vi "FTW-Messenger-Actor-Request.vi"(0 "Messenger":refnum<class "FTW-Messenger-Actor.lvclass">, 5 "Parameter":string, 7 "Payload":variant, 11 "error in":errorcluster) -> (4 "Messenger out":refnum<class "FTW-Messenger-Actor.lvclass">, 15 "error out":errorcluster)   [LabVIEW 2013, in "FTW-Messenger-Actor.lvclass"]
uses:
  FTW-Messenger-Actor.lvclass
  Message.Actor/FTW-Message-Actor.lvclass
  Messenger/FTW-Messenger.lvclass
panel:
  # "Inputs"
  # "Outputs"
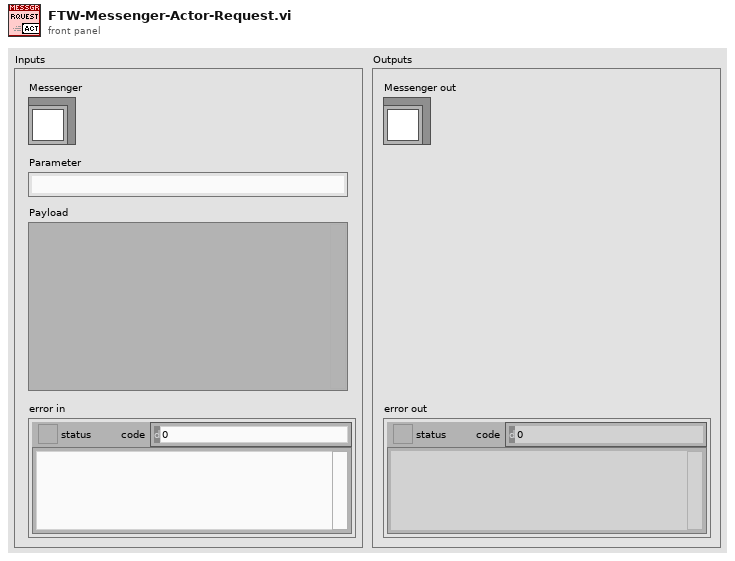
[diagram p1: front panel]
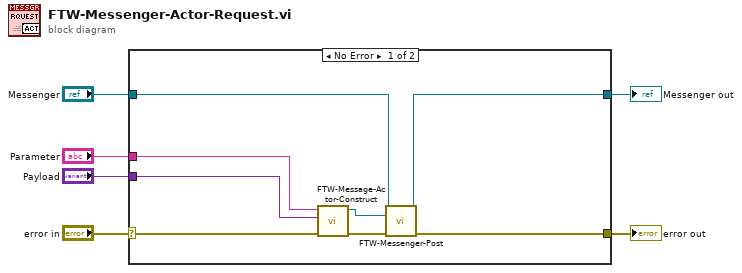
[diagram p0: block diagram]
diagram:
  n1 = case shown="No Error" "error in" {
    selector: "error in" -> [w11 w16]
    tunnel: [w12 w16] -> w5
    tunnel: [w13 w15] -> w6
    tunnel: "Messenger" -> [w14 w15]
    tunnel: "Parameter" -> [w9 _]
    tunnel: "Payload" -> [w8 _]
    frame No Error {
      n2 = call "FTW-Message-Actor-Construct.vi"("error in"=w11, "Payload"=w8, "Parameter"=w9) -> ("error out"=w10:errorcluster, "Actor Message"=w7:refnum<class "FTW-Message-Actor.lvclass">)  [unwired: 7 in]
      n3 = call "FTW-Messenger-Post.vi"("Messenger"=w14, "Message"=w7, "error in"=w10) -> ("Messenger out"=w13:refnum<class "FTW-Messenger-Actor.lvclass">, "error out"=w12:errorcluster)  [unwired: 11 in]
    }
    frame Error {
    }
  }
  "Messenger out" <- w6
  "error out" <- w5
